vi "check_array_with_empty_strings.vi"(10 "String array":string[](array[string])) -> (2 "array with empty strings?":bool)   [LabVIEW 2015]
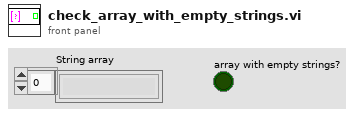
[diagram p1: front panel]
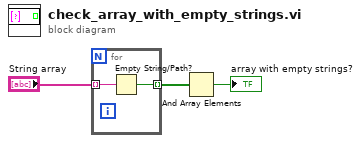
[diagram p0: block diagram]
diagram:
  n1 = for {
    tunnel: "String array" -> [w5] mode=indexing
    tunnel: [w4] -> w2 mode=indexing
    n2 = Empty String/Path?(string/path=w5) -> (empty?=w4:bool)
  }
  n3 = And Array Elements(Boolean array=w2) -> (logical AND=→"array with empty strings?":bool)
